vi "State.vi"() -> ()   [LabVIEW 2015]
panel:
  in  "stop":bool
  out "Boolean 2":bool
  in  "Boolean":bool
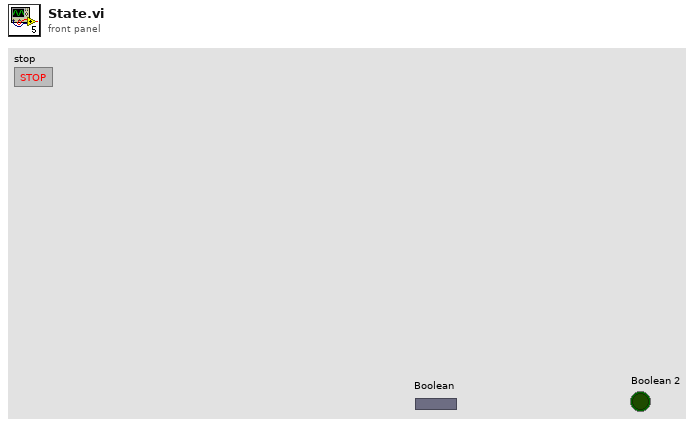
[diagram p1: front panel]
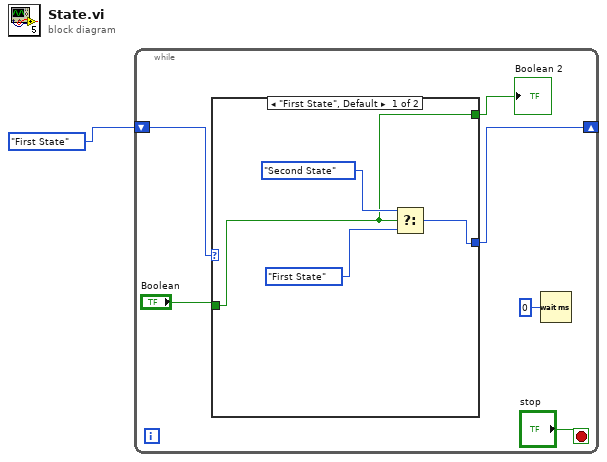
[diagram p0: block diagram]
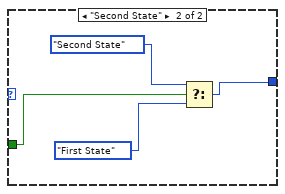
[diagram p2: hidden frame]
diagram:
  n1 = while {
    shift-right: [w7] -> _
    shift-left: enum16{"First State", "Second State"}."First State" -> [w6]
    stop <- "stop" stop-if-true
    n2 = case shown="\"First State\", Default" w6 {
      tunnel: [w9 w13] -> w7
      tunnel: "Boolean" -> [w8 w12]
      tunnel: [w8 _] -> w4
      frame "First State", Default {
        n3 = Select(t=enum16{"First State", "Second State"}."Second State", s=w8, f=enum16{"First State", "Second State"}."First State") -> (s? t:f=w9:enum16{"First State", "Second State"})
      }
      frame "Second State" {
        n4 = Select(t=enum16{"First State", "Second State"}."Second State", s=w12, f=enum16{"First State", "Second State"}."First State") -> (s? t:f=w13:enum16{"First State", "Second State"})
      }
    }
    "Boolean 2" <- w4
    n5 = Wait (ms)(milliseconds to wait=u32 0) -> ()  [unwired: 1 out]
  }
